vi "auto info.vi"(1 "Autonomous Mode":T1(radio)=enum."Autonomous 1 (Drive)") -> (0 "About Selected Auto Mode":string)   [LabVIEW 2014]
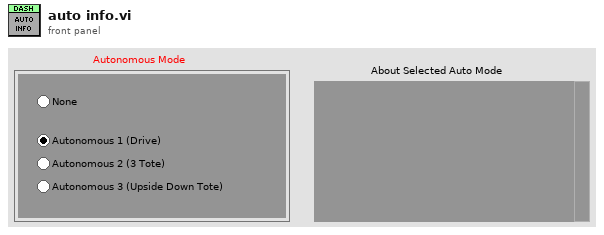
[diagram p1: front panel]
types:
  T1 = enum32{"None", "Autonomous 1 (Drive)", "Autonomous 2 (3 Tote)", "Autonomous 3 (Upside Down Tote)"}
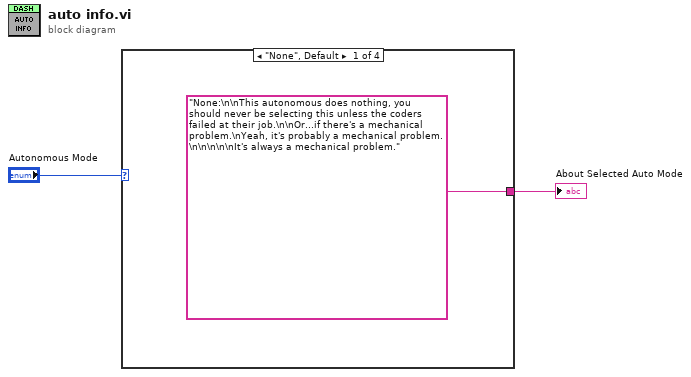
[diagram p0: block diagram]
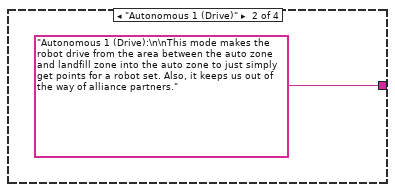
[diagram p2: hidden frame]
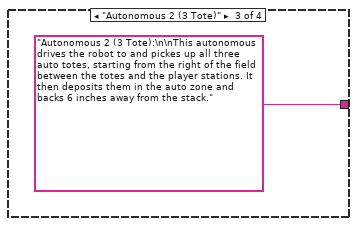
[diagram p3: hidden frame]
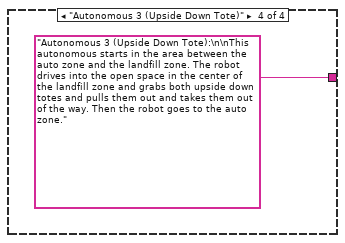
[diagram p4: hidden frame]
diagram:
  n1 = case shown="\"None\", Default" "Autonomous Mode" {
    tunnel: ["None:\n\nThis autonomous does nothing, you should never be selecting this unless the coders failed at their job.\n\nOr...if there's a mechanical problem.\nYeah, it's probably a mechanical problem.\n\n\n\n\nIt's always a mechanical problem." "Autonomous 1 (Drive):\n\nThis mode makes the robot drive from the area between the auto zone and landfill zone into the auto zone to just simply get points for a robot set. Also, it keeps us out of the way of alliance partners." "Autonomous 2 (3 Tote):\n\nThis autonomous drives the robot to and pickes up all three auto totes, starting from the right of the field between the totes and the player stations. It then deposits them in the auto zone and backs 6 inches away from the stack." "Autonomous 3 (Upside Down Tote):\n\nThis autonomous starts in the area between the auto zone and the landfill zone. The robot drives into the open space in the center of the landfill zone and grabs both upside down totes and pulls them out and takes them out of the way. Then the robot goes to the auto zone."] -> w1
    frame "None", Default {
    }
    frame "Autonomous 1 (Drive)" {
    }
    frame "Autonomous 2 (3 Tote)" {
    }
    frame "Autonomous 3 (Upside Down Tote)" {
    }
  }
  "About Selected Auto Mode" <- w1
